vi "proj2012.vi"() -> ()   [LabVIEW 2018]
panel:
  out "Enum":T1(ring)
  in  "Start System":bool
  in  "stop":bool
  in  "Temperature":dbl
  in  "Tank Level #2":dbl
  in  "Tank Level #1":dbl
  in  "Feed Tank Level":dbl
  in  "Proximity #2":bool
  in  "Proximity #1":bool
  out "Temperature":dbl
  out "Tank #2":dbl
  out "Tank #1":dbl
  out "Feed Tank Level":dbl
  out "Heater":bool
  out "Conveyor":bool
  out "Drop Valve #2":bool
  out "Drop Valve #1":bool
  out "Feed Valve #2":bool
  out "Feed Valve #1":bool
  out "Pump":bool
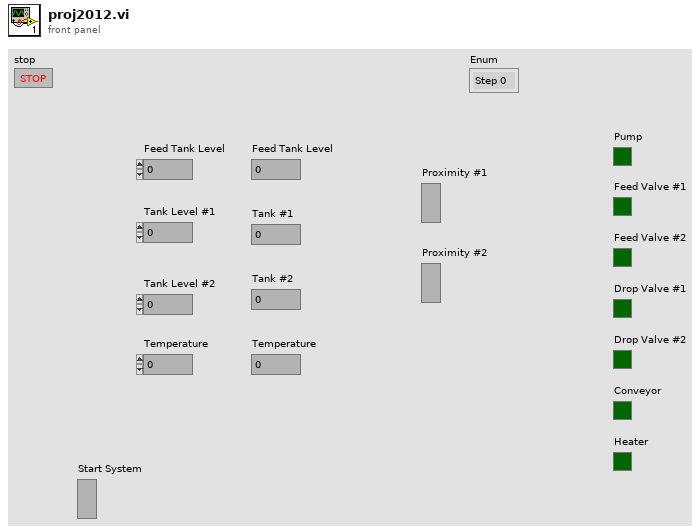
[diagram p1: front panel]
types:
  T1 = enum16{"Step 0", "Step 1", "Step 2", "Step 3", "Step 4", "Step 5", "Step 6", "Step 7"}
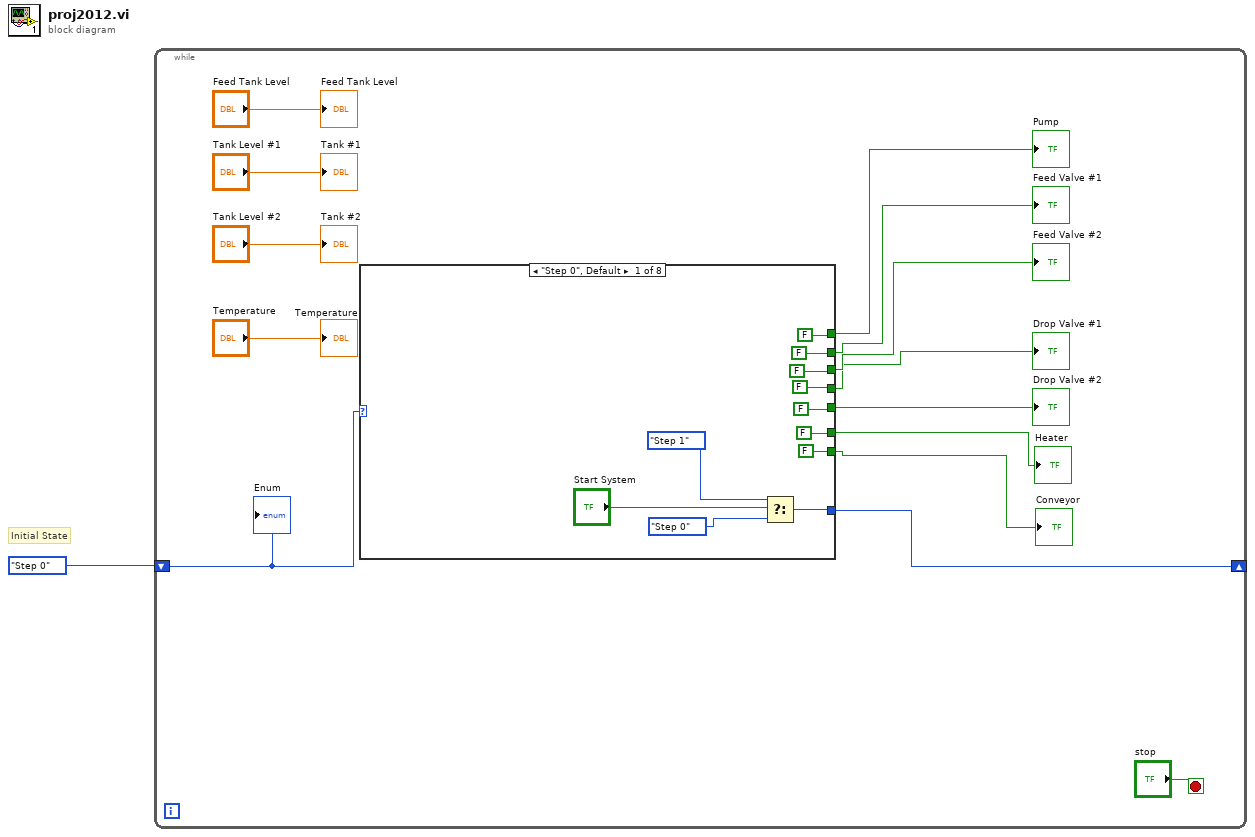
[diagram p0: block diagram]
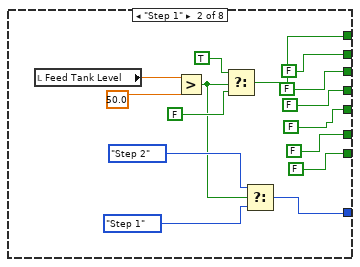
[diagram p2: hidden frame]
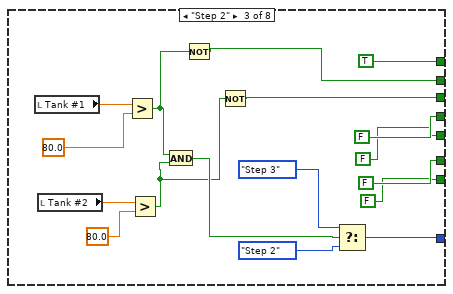
[diagram p3: hidden frame]
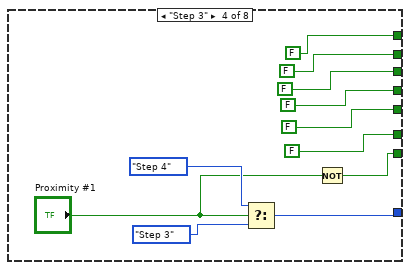
[diagram p4: hidden frame]
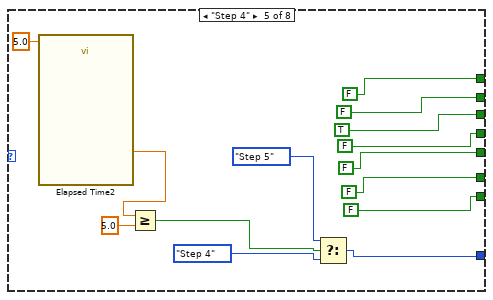
[diagram p5: hidden frame]
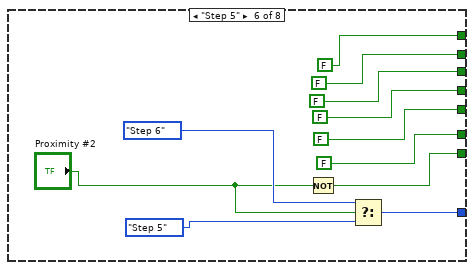
[diagram p6: hidden frame]
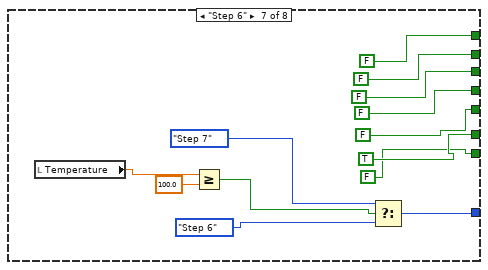
[diagram p7: hidden frame]
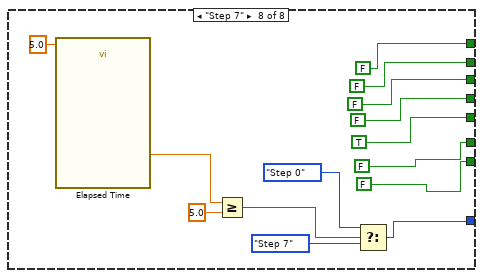
[diagram p8: hidden frame]
diagram:
  # "Initial State"
  n1 = while {
    shift-right: [w2] -> _
    shift-left: T1."Step 0" -> [w3]
    stop <- "stop" stop-if-true
    n2 = case shown="\"Step 0\", Default" w3 {
      tunnel: [FALSE w33 TRUE FALSE FALSE FALSE FALSE FALSE] -> w11
      tunnel: [FALSE FALSE w45 FALSE FALSE FALSE FALSE FALSE] -> w10
      tunnel: [FALSE FALSE w42 FALSE TRUE FALSE FALSE FALSE] -> w9
      tunnel: [FALSE FALSE FALSE FALSE FALSE FALSE FALSE FALSE] -> w8
      tunnel: [FALSE FALSE FALSE FALSE FALSE FALSE FALSE TRUE] -> w7
      tunnel: [FALSE FALSE FALSE FALSE FALSE FALSE TRUE FALSE] -> w6
      tunnel: [FALSE FALSE FALSE w60 FALSE w88 FALSE FALSE] -> w5
      tunnel: [w19 w30 w53 w63 w76 w87 w100 w111] -> w2
      frame "Step 0", Default {
        n3 = Select(t=T1."Step 1", s="Start System", f=T1."Step 0") -> (s? t:f=w19:T1)
      }
      frame "Step 1" {
        n4 = local read "Feed Tank Level"() -> (w36:dbl)
        n5 = Greater?(x=w36, y=50.0) -> (0:w27:bool)
        n6 = Select(t=TRUE, s=w27, f=FALSE) -> (s? t:f=w33:bool)
        n7 = Select(t=T1."Step 2", s=w27, f=T1."Step 1") -> (s? t:f=w30:T1)
      }
      frame "Step 2" {
        n8 = local read "Tank #1"() -> (w50:dbl)
        n9 = local read "Tank #2"() -> (w49:dbl)
        n10 = Greater?(x=w50, y=80.0) -> (0:w44:bool)
        n11 = Greater?(x=w49, y=80.0) -> (0:w43:bool)
        n12 = And(x=w44, y=w43) -> (x .and. y?=w46:bool)
        n13 = Not(x=w44) -> (.not. x?=w45:bool)
        n14 = Not(x=w43) -> (.not. x?=w42:bool)
        n15 = Select(t=T1."Step 3", s=w46, f=T1."Step 2") -> (s? t:f=w53:T1)
      }
      frame "Step 3" {
        n16 = Select(t=T1."Step 4", s="Proximity #1", f=T1."Step 3") -> (s? t:f=w63:T1)
        n17 = Not(x="Proximity #1") -> (.not. x?=w60:bool)
      }
      frame "Step 4" {
        n18 = call "Elapsed Time2"("Time Target (s)"=5.0) -> ("Elapsed Time (s)"=w70:dbl)  [unwired: 11 in, 7 out]
        n19 = Greater Or Equal?(x=w70, y=5.0) -> (x >= y?=w73:bool)
        n20 = Select(t=T1."Step 5", s=w73, f=T1."Step 4") -> (s? t:f=w76:T1)
      }
      frame "Step 5" {
        n21 = Not(x="Proximity #2") -> (.not. x?=w88:bool)
        n22 = Select(t=T1."Step 6", s="Proximity #2", f=T1."Step 5") -> (s? t:f=w87:T1)
      }
      frame "Step 6" {
        n23 = local read "Temperature"() -> (w97:dbl)
        n24 = Greater Or Equal?(x=w97, y=100.0) -> (x >= y?=w96:bool)
        n25 = Select(t=T1."Step 7", s=w96, f=T1."Step 6") -> (s? t:f=w100:T1)
      }
      frame "Step 7" {
        n26 = call "Elapsed Time"("Time Target (s)"=5.0) -> ("Elapsed Time (s)"=w109:dbl)  [unwired: 11 in, 7 out]
        n27 = Greater Or Equal?(x=w109, y=5.0) -> (x >= y?=w110:bool)
        n28 = Select(t=T1."Step 0", s=w110, f=T1."Step 7") -> (s? t:f=w111:T1)
      }
    }
    "Pump" <- w11
    "Feed Valve #1" <- w10
    "Feed Valve #2" <- w9
    "Drop Valve #1" <- w8
    "Drop Valve #2" <- w7
    "Conveyor" <- w5
    "Heater" <- w6
    "Feed Tank Level" <- "Feed Tank Level"
    "Tank #1" <- "Tank Level #1"
    "Tank #2" <- "Tank Level #2"
    "Temperature" <- "Temperature"
    "Enum" <- w3
  }
